vi "Read_Me.vi"() -> ()   [LabVIEW 2011]
uses:
  LED Display.xctl
panel:
  out "LED Display 2":string(xcontrol)="ABC"
  in  "LED Display":string(xcontrol)="NATI +10 "
  # "You can grow and shrink the XControl... if you grow it in the horizontal, it will add rows to the array, but not if you grow it vertically. \n\nIt has a custom runtime menu over the array portion (for Set Text). This means the standard XControl option of \"Show Diagram\" unavailable. To work around this, I've left the custom runtime menu off when the host VI is actually running so that Show Diagram is availble on the XControl. \n\nThe control can display all printable ASCII characters between 1 & 127."
  # "Right click and select \"Set Text\" to set the value of the\nXControls (or wire a value to the FPTerminals  on the block diagram)."
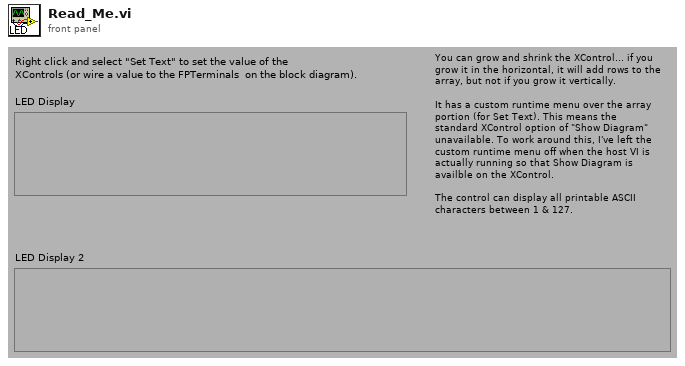
[diagram p1: front panel]
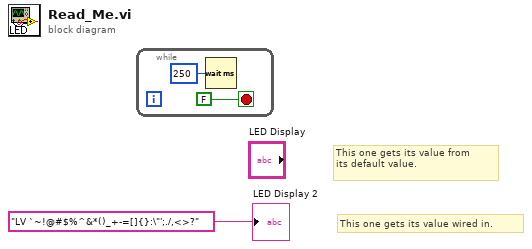
[diagram p0: block diagram]
diagram:
  # "This one gets its value wired in."
  # "This one gets its value from\nits default value."
  n1 = while {
    stop <- FALSE stop-if-true
    n2 = Wait (ms)(milliseconds to wait=u32 250) -> ()  [unwired: 1 out]
  }
  "LED Display 2" <- "LV `~!@#$%^&*()_+-=[]{}:\"';./,<>?" ("LED Display")
